vi "close.vi"(8 "error in (no error)":errorcluster, 11 "toml in":refnum<class "toml.lvclass">) -> (0 "error out":errorcluster)   [LabVIEW 2020, in "toml.lvclass"]
uses:
  toml.lvclass
  toml.lvclass/toml.ctl
  Doc/Doc.lvclass
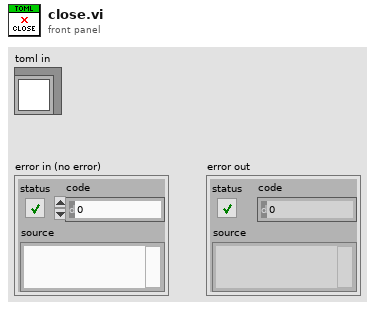
[diagram p1: front panel]
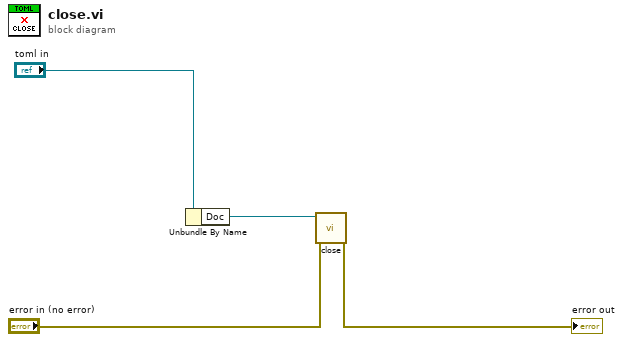
[diagram p0: block diagram]
diagram:
  n1 = Unbundle By Name("toml in") -> ("Doc"=w3:refnum<class "Doc.lvclass">)
  n2 = call "close.vi"("error in (no error)"="error in (no error)", "Doc in"=w3) -> ("error out"=→"error out":errorcluster)  [unwired: 9 in]
